vi "PH_HamamatsuCamera.set Cam Parameters to GUI.vi"(0 "i ref in":refnum<vi>, 5 "error in (no error)":errorcluster) -> (14 "VI out":refnum<vi>, 19 "error out":errorcluster)   [LabVIEW 2014, in "PH_HamamatsuCamera.lvlib"]
uses:
  PH_HamamatsuCamera.lvlib
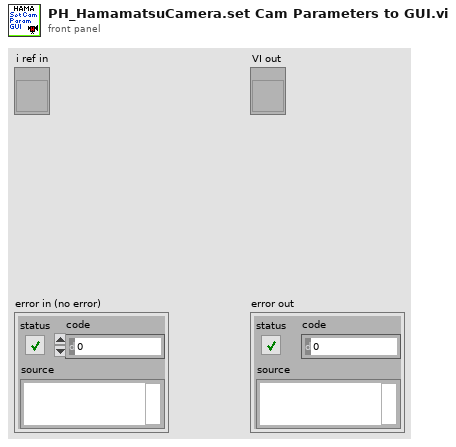
[diagram p1: front panel]
types:
  T1 = typedef "PH_HamamatsuCamera.lvlib/PH_HamamatsuCamera.i attribute.ctl" = cluster{"Gui Refs":cluster{"Camera Details":refnum<vi>, "ROI":refnum<vi>, "Set ROI to Maximum":refnum<vi>, "Trigger Parameters":refnum<vi>, "Brightness":refnum<vi>, "Shutter":refnum<vi>, "Gain":refnum<vi>, "Trigger Timeout":refnum<vi>, "Trigger Polarity":refnum<vi>, "Trigger Mode":refnum<vi>, "Parameters":refnum<vi>, "Set Cam Parameter":refnum<vi>, "Parameter to set":refnum<vi>, "Value to set":refnum<vi>}, "Cam":cluster{"Handle":i32, "Details":cluster{"Model":string, "Camera ID":string, "Firmware":string}, "Buffer Info":cluster{"height":u32, "width":u32, "datatype":u32}}, "H Offset":cluster{"Value":i32, "Minimum":i32, "Maximum":i32, "Increment":i32}, "V Offset":cluster{"Value":i32, "Minimum":i32, "Maximum":i32, "Increment":i32}, "H Width":cluster{"Value":i32, "Minimum":i32, "Maximum":i32, "Increment":i32}, "V Width":cluster{"Value":i32, "Minimum":i32, "Maximum":i32, "Increment":i32}, "Trigger Parameters":T2, "Trigger Timeout":u32, "Parameters":T3[], "Indicees Cam Parameters":cluster{"Brightness":i32, "Shutter":i32, "Gain":i32}, "Wanted Values":cluster{"Trigger Settings":T2[], "ROI":T4[], "Parameter":cluster{"Name":string, "Value":dbl}[]}}
  T2 = typedef "PH_HamamatsuCamera.lvlib/PH_HamamatsuCamera.Trigger Parameter.ctl" = cluster{"Mode":u32, "Polarity":u32, "Times":u32, "Delay":dbl}
  T3 = typedef "PH_HamamatsuCamera.lvlib/PH_HamamatsuCamera.Parameter Set.ctl" = cluster{"Parameter":string, "Value":dbl, "Writable":bool, "Range":cluster{"min":dbl, "max":dbl, "step":dbl}, "Default":dbl, "Value Names":cluster{"Name":string, "Value":dbl}[], "Text Values":bool}
  T4 = typedef "PH_HamamatsuCamera.lvlib/PH_HamamatsuCamera.ROI.ctl" = cluster{"Horizontal Offset":i32, "Vertical Offset":i32, "Horizontal Width":i32, "Vertical Width":i32}
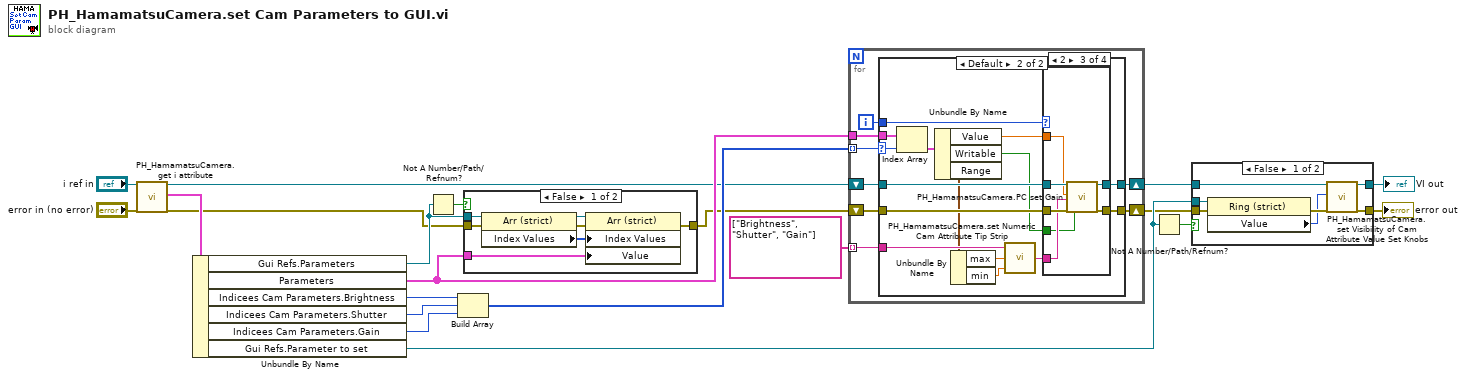
[diagram p0: block diagram]
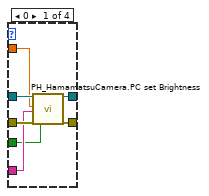
[diagram p3: hidden frame]
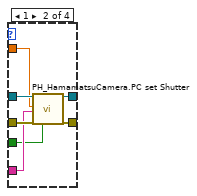
[diagram p4: hidden frame]
diagram:
  n1 = call "PH_HamamatsuCamera.get i attribute.vi"("i ref in"="i ref in", "error in (no error)"="error in (no error)") -> ("i ref out"=w4:refnum<vi>, "i attribute"=w18:T1, "error out"=w15:errorcluster)  [unwired: 15 in]
  n2 = Unbundle By Name(w18) -> ("Gui Refs.Parameters"=w16:refnum<vi>, "Parameters"=w6:T3[], "Indicees Cam Parameters.Brightness"=w14:i32, "Indicees Cam Parameters.Shutter"=w13:i32, "Indicees Cam Parameters.Gain"=w12:i32, "Gui Refs.Parameter to set"=w10:refnum<vi>)
  n3 = Not A Number/Path/Refnum?(number/path/refnum=w16) -> (NaN/Path/Refnum?=w17:bool)
  n4 = Build Array(w14, w13, w12) -> (w5:i32[])
  n5 = case shown="False" w17 {
    tunnel: [w24 w28] -> w3
    tunnel: w6 -> [w21 _]
    tunnel: w15 -> [w27 w28]
    tunnel: w16 -> [w26 _]
    frame False {
      n6 = property class="Arr (strict)"(reference=w26, error in=w27) -> (reference out=w22:refnum<vi>, error out=w25:errorcluster, "Index Values"=w23:u32[])
      n7 = property class="Arr (strict)"(reference=w22, error in=w25, "Index Values"=w23, "Value"=w21) -> (error out=w24:errorcluster)  [unwired: 1 out]
    }
    frame True {
    }
  }
  n8 = for {
    shift-right: [w36] -> w1
    shift-left: w3 -> [w31]
    shift-right: [w34] -> w2
    shift-left: w4 -> [w35]
    tunnel: string[] ["Brightness", "Shutter", "Gain"] -> [w32] mode=indexing
    tunnel: w5 -> [w29] mode=indexing
    tunnel: w6 -> [w30]
    i -> [w33]
    n9 = case shown="Default" w29 {
      selector: w29 -> [_ w41]
      tunnel: [w37 w53] -> w36
      tunnel: w35 -> [w38 w52]
      tunnel: [w38 w51] -> w34
      tunnel: w33 -> [_ w50]
      tunnel: w32 -> [_ w49]
      tunnel: w31 -> [w37 w47]
      tunnel: w30 -> [_ w44]
      frame -1 {
      }
      frame Default {
        n10 = Index Array(array=w44, index=w41) -> (element=w43:T3)
        n11 = Unbundle By Name(w43) -> ("Value"=w40:dbl, "Writable"=w39:bool, "Range"=w42:cluster{"min":dbl, "max":dbl, "step":dbl})
        n12 = Unbundle By Name(w42) -> ("max"=w46:dbl, "min"=w45:dbl)
        n13 = call "PH_HamamatsuCamera.set Numeric Cam Attribute Tip Strip.vi"("Minimum"=w45, "Maximum"=w46, "Attribute"=w49) -> ("Tip Strip"=w48:string)
        n14 = case shown="2" w50 {
          tunnel: w47 -> [w58 w65 w72 w76]
          tunnel: [w55 w62 w69 w76] -> w53
          tunnel: w52 -> [w60 w67 w74 w75]
          tunnel: [w59 w64 w73 w75] -> w51
          tunnel: w40 -> [w57 w66 w71 _]
          tunnel: w48 -> [w56 w63 w70 _]
          tunnel: w39 -> [w54 w61 w68 _]
          frame 0 {
            n15 = call "PH_HamamatsuCamera.PC set Brightness.vi"("i ref in"=w60, "Brightness"=w57, "Tip Strip"=w56, "error in (no error)"=w58, "Brightness writable? (True)"=w54) -> ("i ref out"=w59:refnum<vi>, "error out"=w55:errorcluster)  [unwired: 13 in]
          }
          frame 1 {
            n16 = call "PH_HamamatsuCamera.PC set Shutter.vi"("i ref in"=w67, "Shutter"=w66, "Tip Strip"=w63, "error in (no error)"=w65, "Shutter writable? (True)"=w61) -> ("i ref out"=w64:refnum<vi>, "error out"=w62:errorcluster)  [unwired: 13 in]
          }
          frame 2 {
            n17 = call "PH_HamamatsuCamera.PC set Gain.vi"("i ref in"=w74, "Gain"=w71, "Tip Strip"=w70, "error in (no error)"=w72, "Gain writable? (True)"=w68) -> ("i ref out"=w73:refnum<vi>, "error out"=w69:errorcluster)  [unwired: 13 in]
          }
          frame Default {
          }
        }
      }
    }
  }
  n18 = Not A Number/Path/Refnum?(number/path/refnum=w10) -> (NaN/Path/Refnum?=w11:bool)
  n19 = case shown="False" w11 {
    tunnel: w2 -> [w83 w85]
    tunnel: [w82 w85] -> w9
    tunnel: w1 -> [w81 w84]
    tunnel: [w80 w84] -> w8
    tunnel: w10 -> [w78 _]
    frame False {
      n20 = property class="Ring (strict)"(reference=w78, error in=w81) -> (error out=w79:errorcluster, "Value"=w77:u32)  [unwired: 1 out]
      n21 = call "PH_HamamatsuCamera.set Visibility of Cam Attribute Value Set Knobs.vi"("VI in"=w83, "Parameter"=w77, "error in (no error)"=w79) -> ("VI out"=w82:refnum<vi>, "error out"=w80:errorcluster)  [unwired: 15 in]
    }
    frame True {
    }
  }
  "VI out" <- w9
  "error out" <- w8
